vi "FS Sketch Functions.vi"(6 "Sketch/Body #":i32=1, 7 "Feature In":string="FeatureScript 1247;\nimport(path : \"onshape/std/geometry.fs\", version : \"1247.0\");\n\nannotation { \"Feature Type Name\" : \"LabVIEW Feature\" }\nexport const myFeature = defineFeature(function(context is Context, id is Id, definition is map)\n    precondition\n    {\n        // Define the parameters of the feature type\n    }\n    {\n        // Define the function's action\n    });", 8 "text":T1={"left"=0, "top"=2, "right"=4, "bottom"=0, "String"="Text"}, 9 "elipse":T2={"center x"=0, "center y"=0, "major radius"=2, "minor radius"=4}, 10 "rect":T3={"left"=0, "top"=0, "right"=3, "bottom"=4}, 11 "Sketch Shape":T4) -> (3 "Feature Out":string="FeatureScript 1247;\nimport(path : \"onshape/std/geometry.fs\", version : \"1247.0\");\n\nannotation { \"Feature Type Name\" : \"LVFeat1\" }\nexport const myFeature = defineFeature(function(context is Context, id is Id, definition is map)\n    precondition\n    {\n        // Define the parameters of the feature type\n    }\n    {\n        // Define the function's action\n\nvar sketch1 = newSketch(context, id + \"sketch1\", {\n                \"sketchPlane\" : qCreatedBy(makeId(\"Top\"), EntityType.FACE)\n        });\n        // Create sketch entities here\n        skRectangle(sketch1, \"rectangle1\", {\n                \"firstCorner\" : vector(0, 0) * inch,\n                \"secondCorner\" : vector(3, 4) * inch\n        });\n        \n        skSolve(sketch1);\n    });")   [LabVIEW 2019]
uses:
  Sketch Shapes.ctl
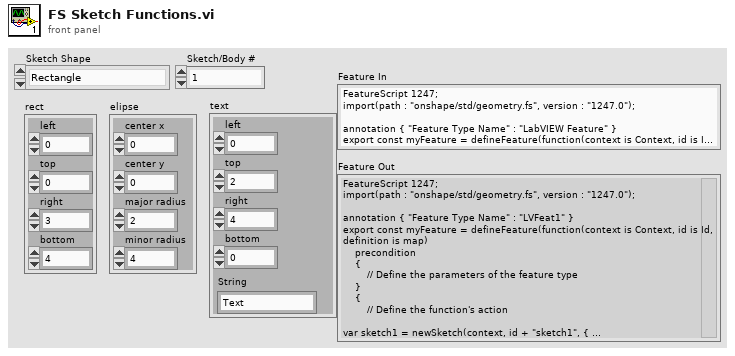
[diagram p1: front panel]
types:
  T1 = cluster{"left":i16, "top":i16, "right":i16, "bottom":i16, "String":string}
  T2 = cluster{"center x":i16, "center y":i16, "major radius":i16, "minor radius":i16}
  T3 = cluster{"left":i16, "top":i16, "right":i16, "bottom":i16}
  T4 = typedef "Sketch Shapes.ctl" = enum16{"Rectangle", "Elipse", "Text"}
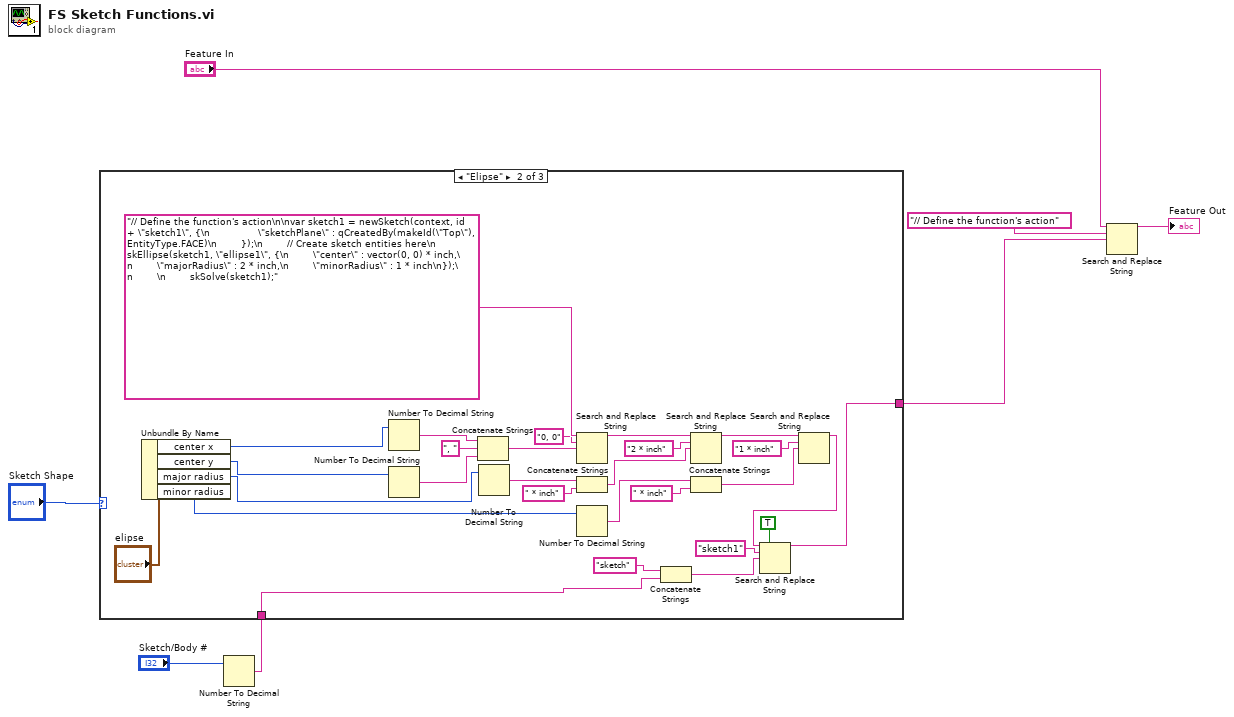
[diagram p0: block diagram]
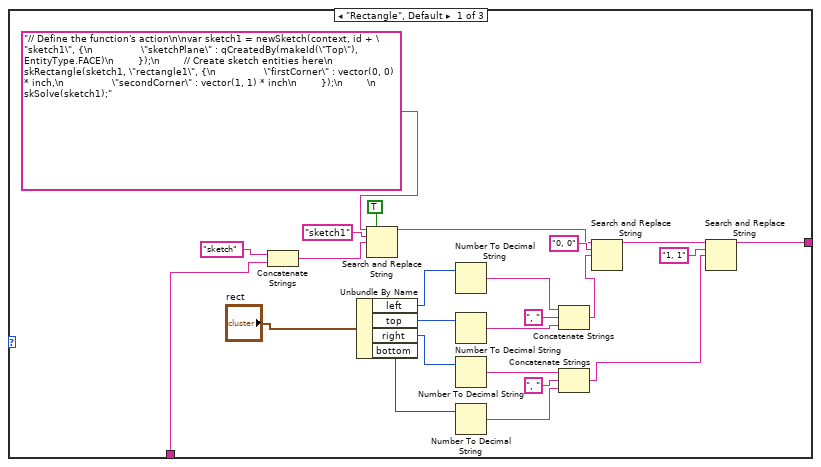
[diagram p2: hidden frame]
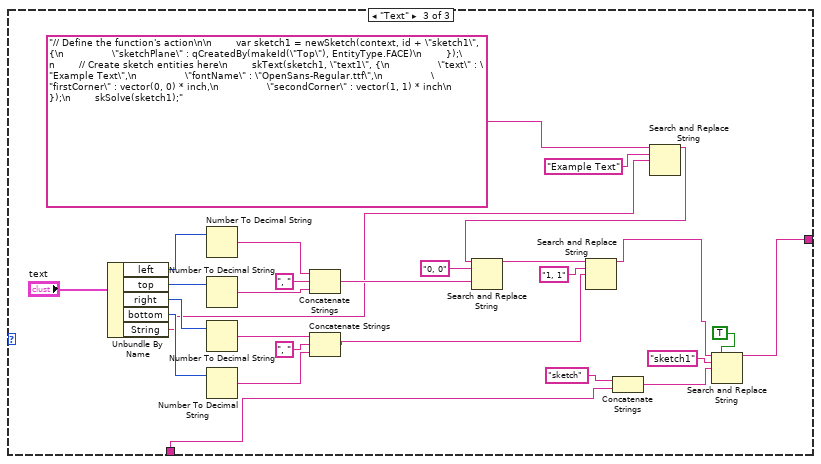
[diagram p3: hidden frame]
diagram:
  n1 = Number To Decimal String(number="Sketch/Body #") -> (decimal integer string=w1:string)  [unwired: 1 in]
  n2 = case shown="\"Elipse\"" "Sketch Shape" {
    tunnel: [w15 w32 w60] -> w6
    tunnel: w1 -> [w11 w34 w62]
    frame "Rectangle", Default {
      n3 = Concatenate Strings("sketch" ("regular expression"), w11) -> (w10:string)
      n4 = Unbundle By Name("rect") -> ("left"=w24:i16, "top"=w23:i16, "right"=w22:i16, "bottom"=w21:i16)
      n5 = Search and Replace String(replace all?=TRUE ("replace all? (F)"), input string="// Define the function's action\n\nvar sketch1 = newSketch(context, id + \"sketch1\", {\n                \"sketchPlane\" : qCreatedBy(makeId(\"Top\"), EntityType.FACE)\n        });\n        // Create sketch entities here\n        skRectangle(sketch1, \"rectangle1\", {\n                \"firstCorner\" : vector(0, 0) * inch,\n                \"secondCorner\" : vector(1, 1) * inch\n        });\n        \n        skSolve(sketch1);", search string="sketch1" ("regular expression"), replace string=w10) -> (result string=w8:string)  [unwired: 4 in, 3 out]
      n6 = Number To Decimal String(number=w24) -> (decimal integer string=w28:string)  [unwired: 1 in]
      n7 = Number To Decimal String(number=w23) -> (decimal integer string=w29:string)  [unwired: 1 in]
      n8 = Number To Decimal String(number=w22) -> (decimal integer string=w31:string)  [unwired: 1 in]
      n9 = Number To Decimal String(number=w21) -> (decimal integer string=w30:string)  [unwired: 1 in]
      n10 = Concatenate Strings(w28, ", " ("regular expression"), w29) -> (w17:string)
      n11 = Concatenate Strings(w31, ", " ("regular expression"), w30) -> (w16:string)
      n12 = Search and Replace String(input string=w8, search string="0, 0" ("regular expression"), replace string=w17) -> (result string=w18:string)  [unwired: 5 in, 3 out]
      n13 = Search and Replace String(input string=w18, search string="1, 1" ("regular expression"), replace string=w16) -> (result string=w15:string)  [unwired: 5 in, 3 out]
    }
    frame "Elipse" {
      n14 = Unbundle By Name("elipse") -> ("center x"=w42:i16, "center y"=w41:i16, "major radius"=w40:i16, "minor radius"=w39:i16)
      n15 = Number To Decimal String(number=w42) -> (decimal integer string=w57:string)  [unwired: 1 in]
      n16 = Number To Decimal String(number=w41) -> (decimal integer string=w55:string)  [unwired: 1 in]
      n17 = Concatenate Strings(w57, ", " ("regular expression"), w55) -> (w54:string)
      n18 = Number To Decimal String(number=w40) -> (decimal integer string=w50:string)  [unwired: 1 in]
      n19 = Search and Replace String(input string="// Define the function's action\n\nvar sketch1 = newSketch(context, id + \"sketch1\", {\n                \"sketchPlane\" : qCreatedBy(makeId(\"Top\"), EntityType.FACE)\n        });\n        // Create sketch entities here\n       skEllipse(sketch1, \"ellipse1\", {\n        \"center\" : vector(0, 0) * inch,\n        \"majorRadius\" : 2 * inch,\n        \"minorRadius\" : 1 * inch\n});\n        \n        skSolve(sketch1);" ("string"), search string="0, 0" ("regular expression"), replace string=w54) -> (result string=w52:string)  [unwired: 5 in, 3 out]
      n20 = Concatenate Strings(w50, " * inch" ("regular expression")) -> (w49:string)
      n21 = Number To Decimal String(number=w39) -> (decimal integer string=w46:string)  [unwired: 1 in]
      n22 = Concatenate Strings("sketch" ("regular expression"), w34) -> (w35:string)
      n23 = Search and Replace String(input string=w52, search string="2 * inch" ("regular expression"), replace string=w49) -> (result string=w51:string)  [unwired: 5 in, 3 out]
      n24 = Concatenate Strings(w46, " * inch" ("regular expression")) -> (w44:string)
      n25 = Search and Replace String(input string=w51, search string="1 * inch" ("regular expression"), replace string=w44) -> (result string=w33:string)  [unwired: 5 in, 3 out]
      n26 = Search and Replace String(replace all?=TRUE ("replace all? (F)"), input string=w33, search string="sketch1" ("regular expression"), replace string=w35) -> (result string=w32:string)  [unwired: 4 in, 3 out]
    }
    frame "Text" {
      n27 = Unbundle By Name("text") -> ("left"=w75:i16, "top"=w76:i16, "right"=w79:i16, "bottom"=w80:i16, "String"=w67:string)
      n28 = Number To Decimal String(number=w75) -> (decimal integer string=w77:string)  [unwired: 1 in]
      n29 = Number To Decimal String(number=w76) -> (decimal integer string=w78:string)  [unwired: 1 in]
      n30 = Number To Decimal String(number=w79) -> (decimal integer string=w82:string)  [unwired: 1 in]
      n31 = Number To Decimal String(number=w80) -> (decimal integer string=w81:string)  [unwired: 1 in]
      n32 = Concatenate Strings(w77, ", " ("regular expression"), w78) -> (w85:string)
      n33 = Concatenate Strings(w82, ", " ("regular expression"), w81) -> (w84:string)
      n34 = Concatenate Strings("sketch" ("regular expression"), w62) -> (w66:string)
      n35 = Search and Replace String(input string="// Define the function's action\n\n        var sketch1 = newSketch(context, id + \"sketch1\", {\n                \"sketchPlane\" : qCreatedBy(makeId(\"Top\"), EntityType.FACE)\n        });\n        // Create sketch entities here\n        skText(sketch1, \"text1\", {\n                \"text\" : \"Example Text\",\n                \"fontName\" : \"OpenSans-Regular.ttf\",\n                \"firstCorner\" : vector(0, 0) * inch,\n                \"secondCorner\" : vector(1, 1) * inch\n        });\n        skSolve(sketch1);" ("search string"), search string="Example Text" ("regular expression"), replace string=w67) -> (result string=w86:string)  [unwired: 5 in, 3 out]
      n36 = Search and Replace String(input string=w86, search string="0, 0" ("regular expression"), replace string=w85) -> (result string=w83:string)  [unwired: 5 in, 3 out]
      n37 = Search and Replace String(input string=w83, search string="1, 1" ("regular expression"), replace string=w84) -> (result string=w61:string)  [unwired: 5 in, 3 out]
      n38 = Search and Replace String(replace all?=TRUE ("replace all? (F)"), input string=w61, search string="sketch1" ("regular expression"), replace string=w66) -> (result string=w60:string)  [unwired: 4 in, 3 out]
    }
  }
  n39 = Search and Replace String(input string="Feature In", search string="// Define the function's action", replace string=w6) -> (result string=→"Feature Out":string)  [unwired: 5 in, 3 out]
